vi "ep_Get EN50160 Signal Level.vi"(0 "signaling frequency [Hz]":dbl=216.66, 5 "nominal voltage [V]":dbl=230.0) -> (4 "signal level [%]":dbl format="%.2f", 6 "signal level [V]":dbl format="%.2f")   [LabVIEW 2011, in "NI_EP_Power Quality.lvlib"]
uses:
  <vilib>/addons/Electrical Power/PQ/NI_EP_Power Quality.lvlib
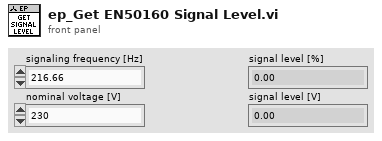
[diagram p1: front panel]
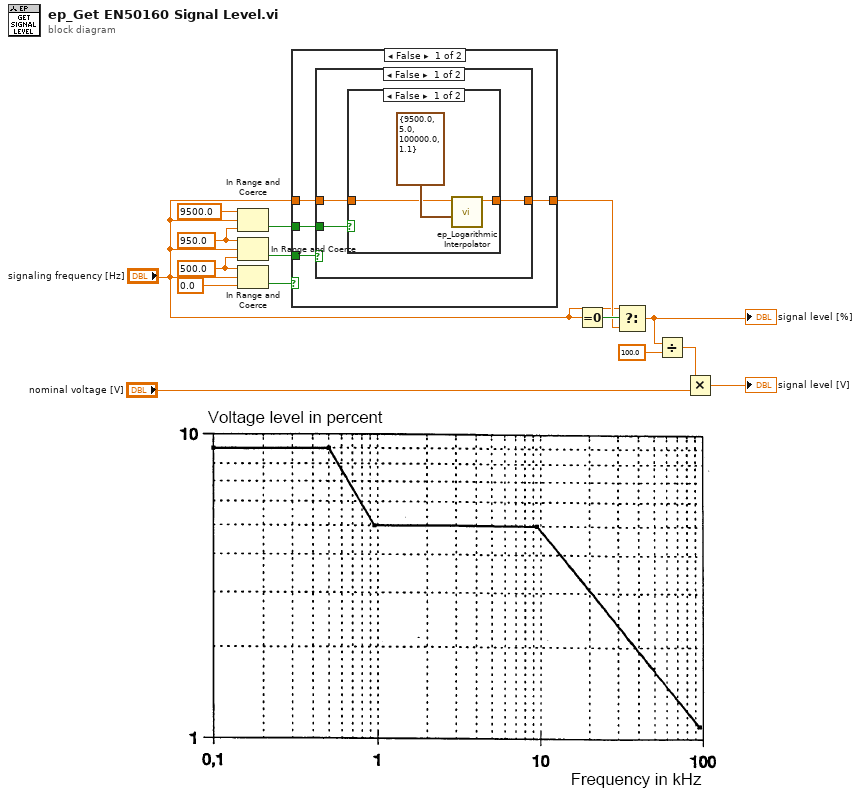
[diagram p0: block diagram]
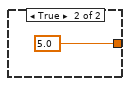
[diagram p2: hidden frame]
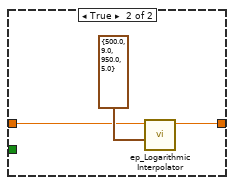
[diagram p3: hidden frame]
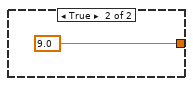
[diagram p4: hidden frame]
diagram:
  w13 = 950.0 ("upper limit")
  w14 = 500.0 ("upper limit")
  n1 = In Range and Coerce(upper limit=9500.0, x="signaling frequency [Hz]", lower limit=w13) -> (In Range?=w10:bool)  [unwired: 1 out]
  n2 = In Range and Coerce(upper limit=w13, x="signaling frequency [Hz]", lower limit=w14) -> (In Range?=w11:bool)  [unwired: 1 out]
  n3 = In Range and Coerce(upper limit=w14, x="signaling frequency [Hz]", lower limit=0.0) -> (In Range?=w12:bool)  [unwired: 1 out]
  n4 = case shown="False" w12 {
    tunnel: w11 -> [w19 _]
    tunnel: w10 -> [w18 _]
    tunnel: "signaling frequency [Hz]" -> [w17 _]
    tunnel: [w16 9.0 ("upper limit")] -> w8
    frame False {
      n5 = case shown="False" w19 {
        tunnel: w18 -> [w20 _]
        tunnel: w17 -> [w21 w28]
        tunnel: [w22 w27] -> w16
        frame False {
          n6 = case shown="False" w20 {
            tunnel: [w23 5.0 ("upper limit")] -> w22
            tunnel: w21 -> [w24 _]
            frame False {
              n7 = call <vilib>:"ep_Logarithmic Interpolator.vi"("points"=cluster{"x1":dbl, "y1":dbl, "x2":dbl, "y2":dbl} {"x1"=9500.0, "y1"=5.0, "x2"=100000.0, "y2"=1.1}, "x"=w24) -> ("y"=w23:dbl)  [unwired: 9 in]
            }
            frame True {
            }
          }
        }
        frame True {
          n8 = call <vilib>:"ep_Logarithmic Interpolator.vi"("points"=cluster{"x1":dbl, "y1":dbl, "x2":dbl, "y2":dbl} {"x1"=500.0, "y1"=9.0, "x2"=950.0, "y2"=5.0}, "x"=w28) -> ("y"=w27:dbl)  [unwired: 9 in]
        }
      }
    }
    frame True {
    }
  }
  n9 = Equal To 0?(x="signaling frequency [Hz]") -> (x = 0?=w9:bool)
  n10 = Select(t="signaling frequency [Hz]", s=w9, f=w8) -> (s? t:f=w7:dbl)
  "signal level [%]" <- w7
  n11 = Divide(x=w7, y=100.0) -> (x/y=w5:dbl)
  n12 = Multiply(x=w5, y="nominal voltage [V]") -> (x*y=→"signal level [V]":dbl)
